vi "ParseMsg.vi"(8 "error in (no error)":errorcluster, 10 "ToParse":string, 11 "MC-ExternClientInterface in":refnum<class "MC-ExternClientInterface.lvclass">) -> (0 "error out":errorcluster, 3 "MC-ExternClientInterface out":refnum<class "MC-ExternClientInterface.lvclass">)   [LabVIEW 2020, in "MC-ExternClient.lvlib" / "MC-ExternClientInterface.lvclass"]
uses:
  MC-ExternClientInterface.lvclass
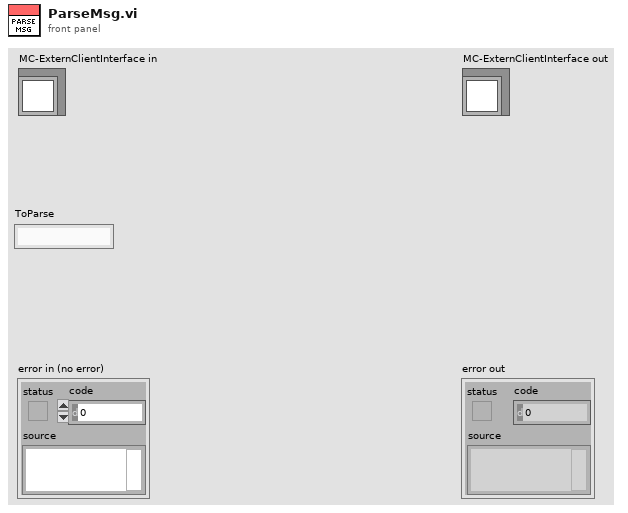
[diagram p1: front panel]
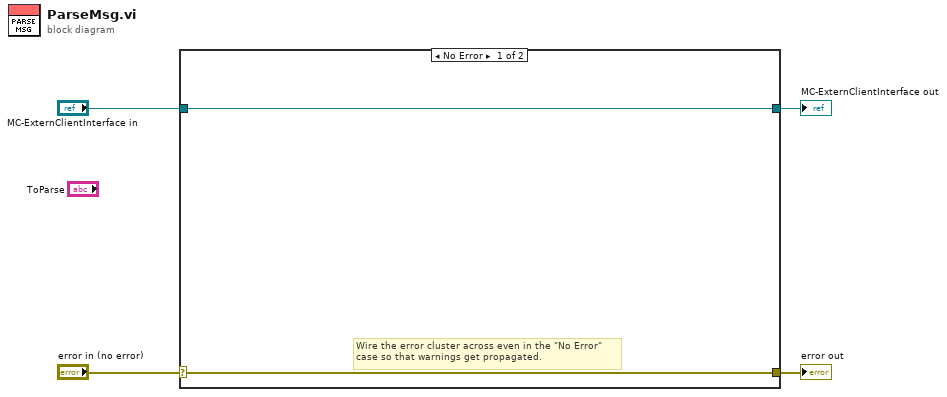
[diagram p0: block diagram]
diagram:
  n1 = case shown="No Error" "error in (no error)" {
    selector: "error in (no error)" -> [w5 w8]
    tunnel: [w5 w8] -> w3
    tunnel: [w6 w7] -> w1
    tunnel: "MC-ExternClientInterface in" -> [w6 w7]
    frame No Error {
      # "Wire the error cluster across even in the \"No Error\"\ncase so that warnings get propagated."
    }
    frame Error {
    }
  }
  "error out" <- w3
  "MC-ExternClientInterface out" <- w1
